vi "AprilTag Target Package Test Code.vi"() -> ()   [LabVIEW 2023]
uses:
  Camera Info.ctl
  State Machine/AprialTag Main Cluster.ctl
  State Machine/AprialTag States.ctl
  <vilib>/vision/Image Controls.llb/IMAQ Image.ctl
  Steam Type.ctl
  Camera Set Up/Event Setup Types.ctl
  <vilib>/Utility/config.llb/Read Key (String).vi
  <vilib>/Utility/config.llb/Write Key (String).vi
  <vilib>/Utility/config.llb/NI_LVConfig.lvlib
panel:
  in  "Main":enum32{"Page 1", "Page 2"}(tab)
  out "Target Pitch":dbl[](array[numeric]) caption="Tag Pitch (deg)" format="%.1f"
  out "Target Roll":dbl[](array[numeric]) caption="Tag Yaw (deg)" format="%.1f"
  out "Tag ID":dbl[](array[numeric]) caption="Tag Number"
  out "Image":T1(plugin-control)
  in  "Camera Name":string="cam0"
  in  "Settings":bool
  in  "Save":bool
  in  "Tools":bool
  out "AprilTag Fps":dbl format="%#.0f"
  out "Distance":dbl[](array[numeric]) caption="Tag Distance (in)" format="%.1f"
  out "Angle":dbl[](array[numeric]) caption="Center Angle (deg)" format="%.1f"
  in  "Home":bool
  in  "FOV":dbl=68.5
  in  "Robot Calibration Cluster":T2={"Camera Height on robot (in)"=9.5, "Camera Angle on the robot (deg)"=2.5, "Camera FOV Top to Bottom View Angle (deg)"=26.5, "Target size (in)"=6.5, "Distance to front of bumper (in)"=9.75} {"Distance to front of bumper (in)" format="%#_13g"; "Target size (in)" format="%#_13g"; "Camera FOV Top to Bottom View Angle (deg)" format="%#_13g"; "Camera Angle on the robot (deg)" format="%#_13g"; "Camera Height on robot (in)" format="%#_13g"}
  # "Edit the camera name to the camera that you are going to use for this target package"
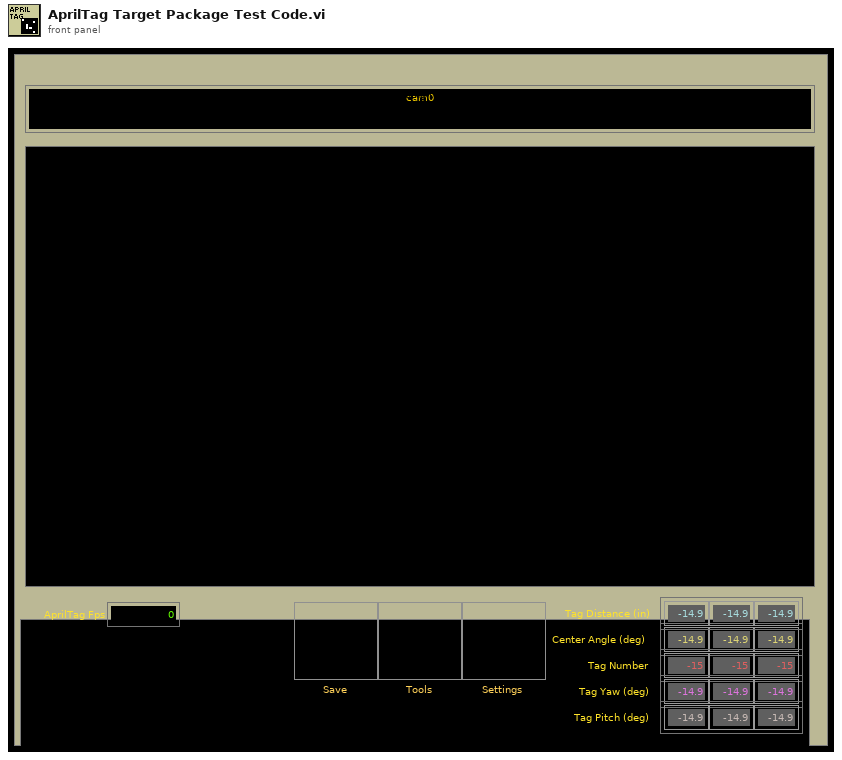
[diagram p1: front panel]
types:
  T1 = typedef "IMAQ Image.ctl" = refnum<image>
  T2 = typedef "Camera Info.ctl" = cluster{"Camera Height on robot (in)":dbl, "Camera Angle on the robot (deg)":dbl, "Camera FOV Top to Bottom View Angle (deg)":dbl, "Target size (in)":dbl, "Distance to front of bumper (in)":dbl}
  T3 = typedef "AprialTag States.ctl" = enum16{"Message Dispatcher", "INI", "Open", "Save", "Exit"}
  T4 = typedef "AprialTag Main Cluster.ctl" = cluster{"AprilTage FIFO":T3[], "Camera Name":string, "AprilTag path":path, "Control Ref's":refnum<vi>[], "Greyscale Mask Image":T1, "Main Image":T1, "Timeout":i32, "EDIT Settings":bool, "Calibration path":path}
  T5 = typedef "Steam Type.ctl" = enum8{"Unknown", "Apriltag", "Algae", "Coral"}
  T6 = typedef "Event Setup Types.ctl" = enum16{"Default", "Camera Loop Started", "Close Settings", "Open Front Panel", "Save Data", "Exit"}
  T7 = typedef "Image Type" = u32
  T8 = cluster{"tag ID":i32, "Center":cluster{"X":dbl, "Y":dbl}, "homography matrix":dbl[], "decision margin":dbl, "Hamming Dist":i32, "corner points":cluster{"X":dbl, "Y":dbl}[], "Tag Family":string}[]
  T9 = typedef "AprilTag Target Fields.ctl" = cluster{"diameter points":cluster{"first point":cluster{"x":dbl, "y":dbl}, "projected point":cluster{"x":dbl, "y":dbl}}, "normalized center":cluster{"x":dbl, "y":dbl}, "Overall Score":dbl, "Distance (ft)":dbl, "Offset Angle":dbl, "Tag corner points":cluster{"X":dbl, "Y":dbl}[], "Tag Center":cluster{"X":dbl, "Y":dbl}, "Tag Yaw":dbl, "Tag Pitch":dbl, "AprilTag Number":i32}
  T10 = typedef "NI_LVConfig.lvlib/Config Data RefNum.ctl" = refnum<k1>
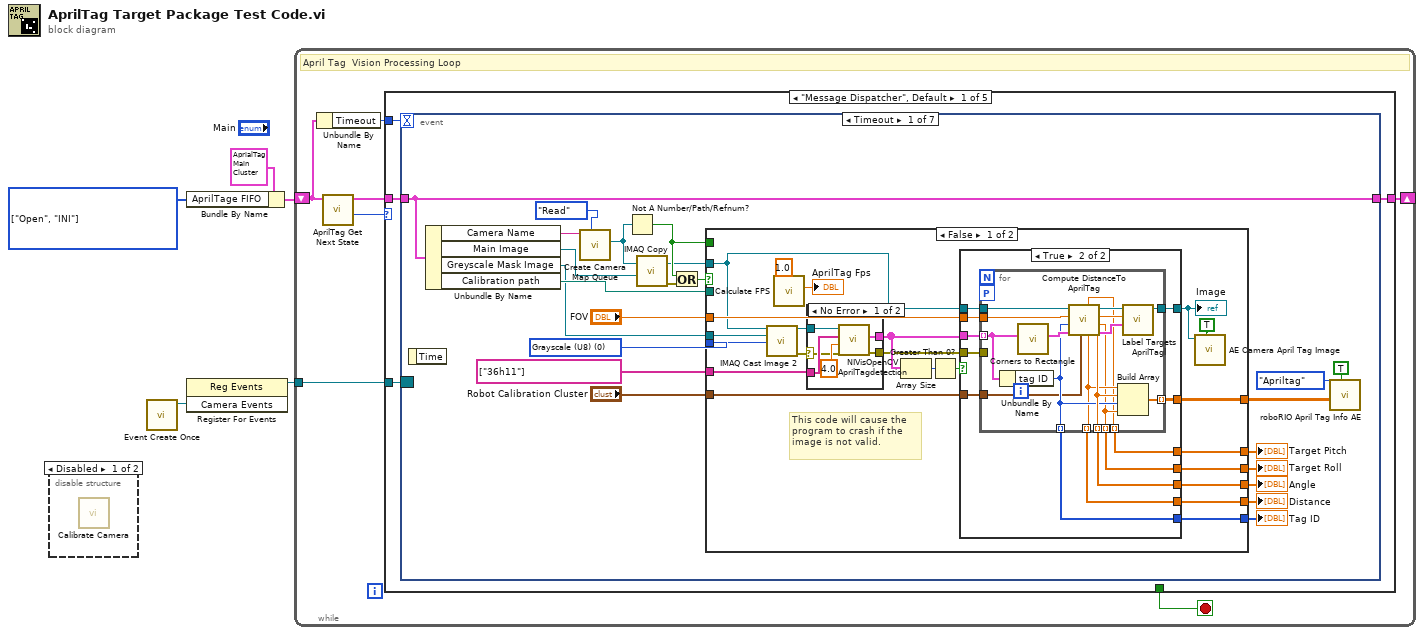
[diagram p0: block diagram]
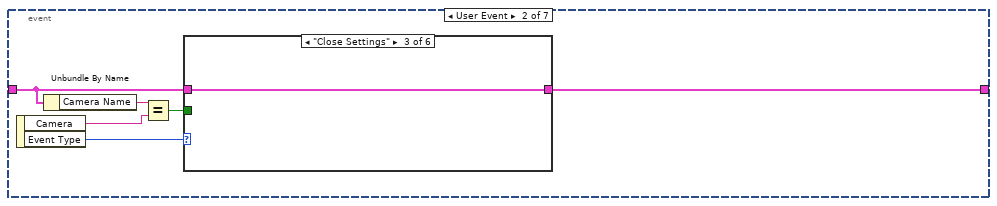
[diagram p6: hidden frame]
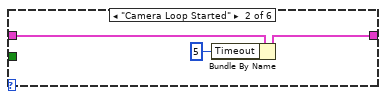
[diagram p8: hidden frame]
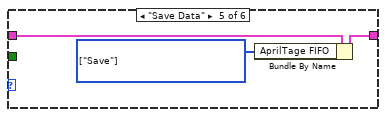
[diagram p10: hidden frame]
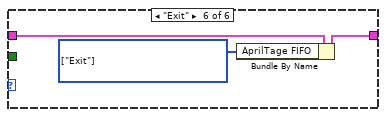
[diagram p11: hidden frame]
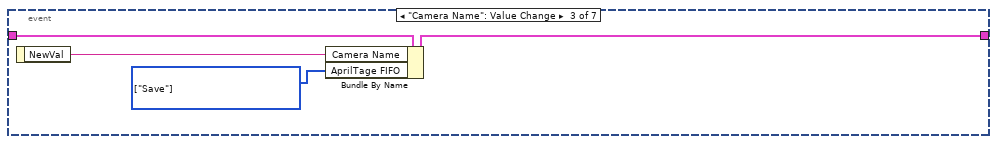
[diagram p12: hidden frame]
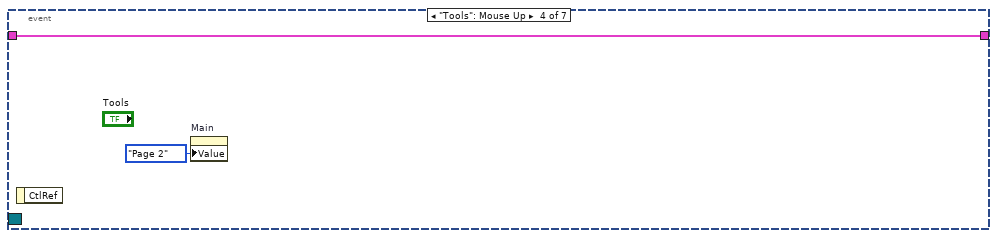
[diagram p13: hidden frame]
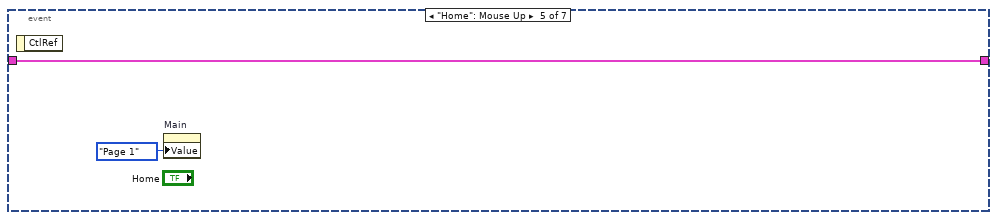
[diagram p14: hidden frame]
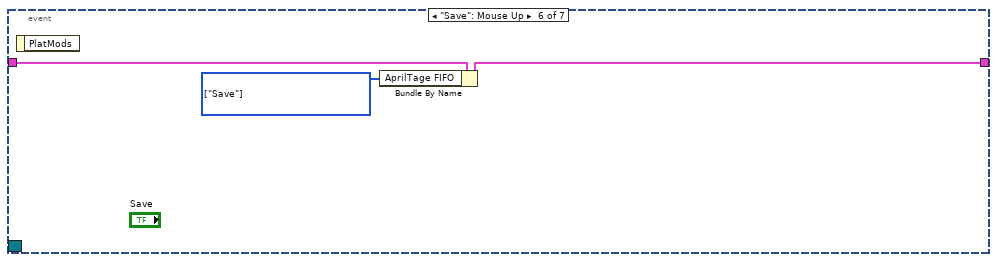
[diagram p15: hidden frame]
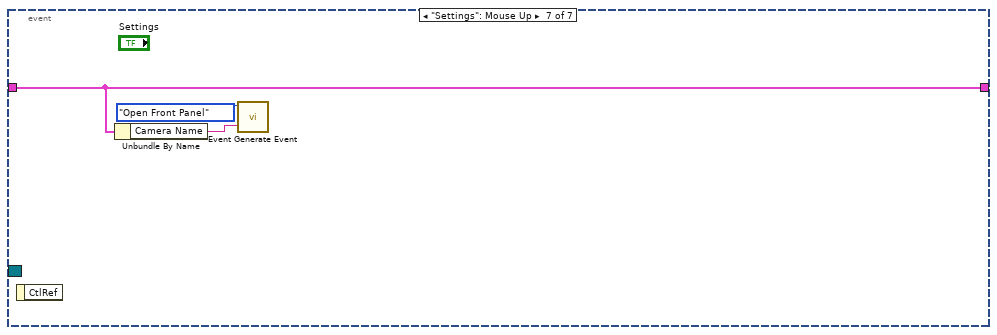
[diagram p16: hidden frame]
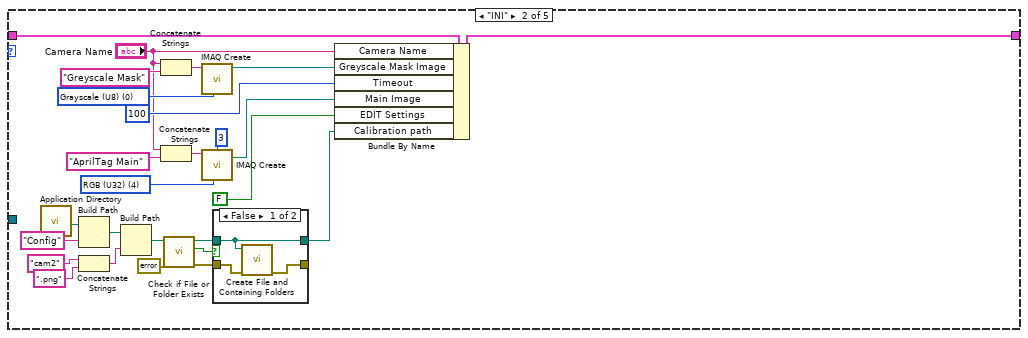
[diagram p17: hidden frame]
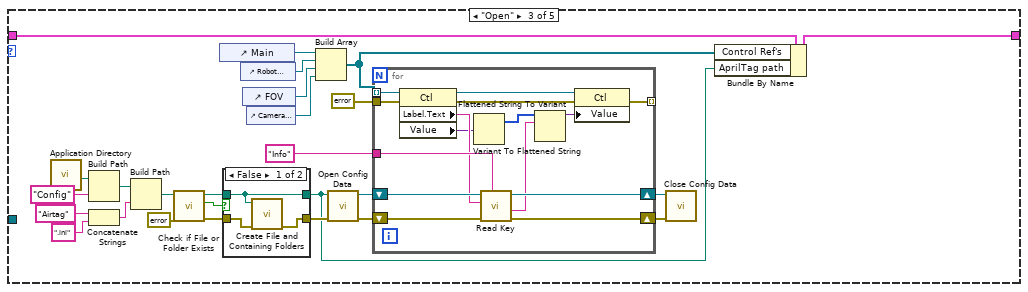
[diagram p19: hidden frame]
diagram:
  w1 = T3[] [enum."Open", enum."INI"] items=["Message Dispatcher", "INI", "Open", "Save", "Exit"] ("AprilTage FIFO")
  n1 = disable-structure shown="Disabled" {
    frame Disabled {
      n2 = call "Calibrate Camera.vi"() -> ()  [unwired: 14 in, 2 out]
    }
    frame Enabled {
    }
  }
  n3 = call "Event Create Once.vi"() -> ("Camera Events"=w5:refnum<user-event>)  [unwired: 10 in, 1 out]
  n4 = Bundle By Name(cluster=T4 {"AprilTage FIFO"=[], "Camera Name"="", "AprilTag path"=path "", "Control Ref's"=[], "Greyscale Mask Image"=refnum, "Main Image"=refnum, "Timeout"=5, "EDIT Settings"=FALSE, "Calibration path"=path ""} ("AprilTag Main Cluster out"), "AprilTage FIFO"=w1) -> (w2:T4)
  n5 = register-events(w5) -> (reference out=w4:refnum<event-registration>)  [unwired: 2 in, 1 out]
  n6 = while {
    tunnel: w4 -> [w12]
    shift-right: [w8] -> _
    shift-left: w2 -> [w6]
    stop <- w11 stop-if-true
    # "April Tag  Vision Processing Loop"
    n7 = Unbundle By Name(w6) -> ("Timeout"=w7:i32)
    n8 = call "AprilTag Get Next State.vi"("AprilTag Main Cluster in"=w6) -> ("Next State"=w9:T3, "AprilTag Main Cluster out"=w10:T4)  [unwired: 9 in]
    n9 = case shown="\"Message Dispatcher\", Default" w9 {
      tunnel: w12 -> [w16 _ _ _ _]
      tunnel: [_ _ _ _ TRUE] -> w11
      tunnel: w10 -> [w14 w153 w170 w208 w225]
      tunnel: [w15 w152 w168 w208 w225] -> w8
      tunnel: w7 -> [w13 _ _ _ _]
      frame "Message Dispatcher", Default {
        n10 = event shown="[0] Timeout" {
          selector: w16 -> [_ _ _ _ _ _ _]
          dyn-events: _ -> [_ _ _ _ _ _ _]
          timeout: w13 -> [_ _ _ _ _ _ _]
          tunnel: w14 -> [w39 w99 w117 w118 w120 w124 w126]
          tunnel: [w39 w101 w116 w118 w120 w123 w126] -> w15
          event Timeout {
            w34 = T7 0 items=["Grayscale (U8)", "Grayscale (I16)", "Grayscale (SGL)", "Complex (CSG)", "RGB (U32)", "HSL (U32)", "RGB (U64)", "Grayscale (U16)"] ("Image Type")
            n11 = event-data() -> ()  [unwired: 1 in, 1 out]
            n12 = Unbundle By Name(w39) -> ("Camera Name"=w23:string, "Main Image"=w17:T1, "Greyscale Mask Image"=w18:T1, "Calibration path"=w35:path)
            n13 = call "Create Camera Map Queue.vi"("Action"=enum16{"Read", "Write"}."Read", "Camera"=w23) -> ("Image out"=w22:T1)  [unwired: 8 in, 1 out]
            n14 = Not A Number/Path/Refnum?(number/path/refnum=w22) -> (NaN/Path/Refnum?=w30:bool)
            n15 = call "IMAQ Copy"("Image Dst"=w17, "Image Src"=w22) -> ("error out"=w20:errorcluster, "Image Dst Out"=w19:T1)  [unwired: 4 in]
            n16 = Or(x=w30, y=w20) -> (x .or. y?=w21:bool)
            n17 = case shown="False" w21 {
              tunnel: w34 -> [w61 _]
              tunnel: string[] ["36h11"] ("Tag Familys") -> [w60 _]
              tunnel: "FOV" -> [w59 _]
              tunnel: "Robot Calibration Cluster" -> [w58 _]
              tunnel: [w48 _] -> w37
              tunnel: w30 -> [_ _]
              tunnel: w35 -> [_ _]
              tunnel: [w46 _] -> w29
              tunnel: [w45 _] -> w28
              tunnel: [w44 _] -> w27
              tunnel: [w43 _] -> w26
              tunnel: [w42 _] -> w25
              tunnel: w19 -> [w41 _]
              tunnel: w18 -> [w40 _]
              frame False {
                # "This code will cause the program to crash if the image is not valid."
                n18 = call "IMAQ Cast Image 2"("Image Src"=w41, "Image Dst"=w40, "Image Type"=w61) -> ("Image Dst Out"=w57:T1, "error out"=w47:errorcluster)  [unwired: 11 in]
                n19 = call "Calculate FPS.vi"("Frames Processed"=1.0) -> ("Fps"=→"AprilTag Fps":dbl)  [unwired: 10 in]
                n20 = case shown="No Error" w47 {
                  selector: w47 -> [w62 w68]
                  tunnel: w60 -> [w67 _]
                  tunnel: w57 -> [w66 _]
                  tunnel: [w65 _] -> w56
                  tunnel: [w64 w68] -> w53
                  frame No Error {
                    n21 = call "NIVisOpenCV AprilTagdetection.vi"("error in (no error)"=w62, "decimate"=4.0, "Tag Familys"=w67, "Image Src"=w66) -> ("error out"=w64:errorcluster, "Detected Tags"=w65:T8)  [unwired: 4 in, 2 out]
                  }
                  frame Error {
                  }
                }
                n22 = Array Size(array=w56) -> (size(s)=w55:i32)
                n23 = Greater Than 0?(x=w55) -> (x > 0?=w54:bool)
                n24 = case shown="True" w54 {
                  tunnel: w41 -> [w69 w81]
                  tunnel: w56 -> [_ w80]
                  tunnel: [w69 w79] -> w52
                  tunnel: w53 -> [_ w78]
                  tunnel: w59 -> [_ w77]
                  tunnel: w58 -> [_ w76]
                  tunnel: [_ w75] -> w48
                  tunnel: [_ w74] -> w46
                  tunnel: [_ w73] -> w45
                  tunnel: [_ w72] -> w44
                  tunnel: [_ w71] -> w43
                  tunnel: [_ w70] -> w42
                  frame False {
                  }
                  frame True {
                    n25 = for {
                      tunnel: w80 -> [w93] mode=indexing
                      tunnel: w81 -> [w94]
                      tunnel: [w95] -> w79
                      tunnel: w78 -> [_]
                      tunnel: [w87] -> w72 mode=indexing
                      tunnel: [w85] -> w70 mode=indexing
                      tunnel: [w89] -> w71 mode=indexing
                      tunnel: w77 -> [w88]
                      tunnel: w76 -> [w86]
                      tunnel: [w84] -> w73 mode=indexing
                      tunnel: [w83] -> w75 mode=indexing
                      tunnel: [w82] -> w74 mode=indexing
                      workers-P: _ -> [_]
                      n26 = Unbundle By Name(w93) -> ("tag ID"=w87:i32)
                      n27 = call "Corners to Rectangle.vi"("tag info"=w93) -> ("output cluster"=w92:T9)  [unwired: 10 in]
                      n28 = call "Compute DistanceTo AprilTag.vi"("Robot Calibration Cluster"=w86, "results"=w92, "AprilTag Number"=w87, "FOV Left to Right (deg)"=w88, "Image Src"=w94) -> ("results out"=w91:T9, "Target Yaw (deg)"=w84:dbl, "Offset Angle"=w89:dbl, "Image Dst Out"=w90:T1, "Distance from target (in)"=w85:dbl, "Target Pitch (deg)"=w82:dbl)  [unwired: 1 in]
                      n29 = Build Array(w85, w89, w87, w84) -> (w83:dbl[])
                      n30 = call "Label Targets AprilTagl.vi"("results"=w91, "Angle"=w89, "Image in"=w90) -> ("Image out"=w95:T1)  [unwired: 8 in]
                    }
                  }
                }
                "Image" <- w52
                n31 = call "AE Camera April Tag Image.vi"("Update"=TRUE, "Ball Image in"=w52) -> ()  [unwired: 9 in, 1 out]
              }
              frame True {
              }
            }
            "Distance" <- w25
            "Angle" <- w26
            "Tag ID" <- w27
            "Target Roll" <- w28
            "Target Pitch" <- w29
            n32 = call "roboRIO April Tag Info AE.vi"("Update"=TRUE, "Info in"=w37, "Stream Type"=Steam_Type."Apriltag") -> ()  [unwired: 8 in, 1 out]
          }
          event User Event {
            n33 = event-data() -> ("Camera"=w97:string, "Event Type"=w100:T6)  [unwired: 1 in]
            n34 = Unbundle By Name(w99) -> ("Camera Name"=w98:string)
            n35 = Equal?(x=w98, y=w97) -> (x = y?=w96:bool)
            n36 = case shown="\"Close Settings\"" w100 {
              tunnel: w99 -> [w102 w105 w106 w107 w110 w113]
              tunnel: [w102 w104 w106 w107 w109 w112] -> w101
              tunnel: w96 -> [_ _ _ _ _ _]
              frame "Default" {
              }
              frame "Camera Loop Started" {
                n37 = Bundle By Name(cluster=w105, "Timeout"=5) -> (w104:T4)
              }
              frame "Close Settings" {
              }
              frame "Open Front Panel" {
              }
              frame "Save Data" {
                w108 = T3[] [enum."Save"] items=["Message Dispatcher", "INI", "Open", "Save", "Exit"] ("AprilTage FIFO")
                n38 = Bundle By Name(cluster=w110, "AprilTage FIFO"=w108) -> (w109:T4)
              }
              frame "Exit" {
                w111 = T3[] [enum."Exit"] items=["Message Dispatcher", "INI", "Open", "Save", "Exit"] ("AprilTage FIFO")
                n39 = Bundle By Name(cluster=w113, "AprilTage FIFO"=w111) -> (w112:T4)
              }
            }
          }
          event "Camera Name": Value Change {
            w115 = T3[] [enum."Save"] items=["Message Dispatcher", "INI", "Open", "Save", "Exit"] ("AprilTage FIFO")
            n40 = event-data() -> ("NewVal"=w114:string)  [unwired: 1 in]
            n41 = Bundle By Name(cluster=w117, "Camera Name"=w114, "AprilTage FIFO"=w115) -> (w116:T4)
          }
          event "Tools": Mouse Up {
            n42 = event-data() -> ()  [unwired: 1 in, 1 out]
            n43 = property on="Main" class="TabCtl (strict)"("Value"=enum32{"Page 1", "Page 2"}."Page 2" ("Main")) -> ()  [unwired: 2 in, 2 out]
          }
          event "Home": Mouse Up {
            n44 = event-data() -> ()  [unwired: 1 in, 1 out]
            n45 = property on="Main" class="TabCtl (strict)"("Value"=enum32{"Page 1", "Page 2"}."Page 1" ("Main")) -> ()  [unwired: 2 in, 2 out]
          }
          event "Save": Mouse Up {
            w122 = T3[] [enum."Save"] items=["Message Dispatcher", "INI", "Open", "Save", "Exit"] ("AprilTage FIFO")
            n46 = event-data() -> ()  [unwired: 1 in, 1 out]
            n47 = Bundle By Name(cluster=w124, "AprilTage FIFO"=w122) -> (w123:T4)
          }
          event "Settings": Mouse Up {
            n48 = event-data() -> ()  [unwired: 1 in, 1 out]
            n49 = Unbundle By Name(w126) -> ("Camera Name"=w125:string)
            n50 = call "Event Generate Event.vi"("Camera Name"=w125, "Event Type"=Event_Setup_Types."Open Front Panel") -> ()  [unwired: 10 in]
          }
        }
      }
      frame "INI" {
        w146 = T7 4 items=["Grayscale (U8)", "Grayscale (I16)", "Grayscale (SGL)", "Complex (CSG)", "RGB (U32)", "HSL (U32)", "RGB (U64)", "Grayscale (U16)"] ("Image Type")
        w149 = T7 0 items=["Grayscale (U8)", "Grayscale (I16)", "Grayscale (SGL)", "Complex (CSG)", "RGB (U32)", "HSL (U32)", "RGB (U64)", "Grayscale (U16)"] ("Image Type")
        n51 = call <vilib>:"Application Directory.vi"() -> ("Application Directory"=w137:path)
        n52 = Build Path(base path=w137, name or relative path="Config") -> (appended path=w135:path)
        n53 = Concatenate Strings("cam2" ("string"), ".png" ("name or relative path")) -> (w139:string)
        n54 = Build Path(base path=w135, name or relative path=w139) -> (appended path=w134:path)
        n55 = Concatenate Strings("Camera Name", "Greyscale Mask" ("string")) -> (w150:string)
        n56 = Concatenate Strings("Camera Name", "AprilTag Main" ("string")) -> (w145:string)
        n57 = call <vilib>:"Check if File or Folder Exists.vi"("error in (no error)"=errorcluster {"status"=FALSE, "code"=0, "source"=""}, "path"=w134) -> ("error out"=w131:errorcluster, "file or folder exists?"=w132:bool, "dup path"=w133:path)  [unwired: 7 in]
        n58 = call "IMAQ Create"("Image Name"=w150, "Image Type"=w149) -> ("New Image"=w148:T1)  [unwired: 2 in, 2 out]
        n59 = call "IMAQ Create"("Border Size"=3, "Image Name"=w145, "Image Type"=w146) -> ("New Image"=w143:T1)  [unwired: 1 in, 2 out]
        n60 = case shown="False" w132 {
          tunnel: [w156 w157] -> _
          tunnel: w133 -> [w155 w158]
          tunnel: [w155 w158] -> w128
          tunnel: w131 -> [w154 w157]
          frame False {
            n61 = call <vilib>:"Create File and Containing Folders.vi"("error in (no error)"=w154, "file path"=w155) -> ("error out"=w156:errorcluster)  [unwired: 8 in, 1 out]
          }
          frame True {
          }
        }
        n62 = Bundle By Name(cluster=w153, "Camera Name"="Camera Name", "Greyscale Mask Image"=w148, "Timeout"=100, "Main Image"=w143, "EDIT Settings"=FALSE, "Calibration path"=w128) -> (w152:T4)
      }
      frame "Open" {
        n63 = call <vilib>:"Application Directory.vi"() -> ("Application Directory"=w173:path)
        n64 = Build Path(base path=w173, name or relative path="Config") -> (appended path=w171:path)
        n65 = Concatenate Strings("Airtag" ("string"), ".ini" ("name or relative path")) -> (w184:string)
        n66 = Build Path(base path=w171, name or relative path=w184) -> (appended path=w164:path)
        n67 = call <vilib>:"Check if File or Folder Exists.vi"("error in (no error)"=errorcluster {"status"=FALSE, "code"=0, "source"=""}, "path"=w164) -> ("error out"=w160:errorcluster, "file or folder exists?"=w162:bool, "dup path"=w163:path)  [unwired: 7 in]
        n68 = control-ref of="Main"() -> (w179:refnum<vi>)
        n69 = case shown="False" w162 {
          tunnel: [w187 w188] -> w174
          tunnel: w163 -> [w186 w189]
          tunnel: [w186 w189] -> w161
          tunnel: w160 -> [w185 w188]
          frame False {
            n70 = call <vilib>:"Create File and Containing Folders.vi"("error in (no error)"=w185, "file path"=w186) -> ("error out"=w187:errorcluster)  [unwired: 8 in, 1 out]
          }
          frame True {
          }
        }
        n71 = control-ref of="Robot Calibration Cluster"() -> (w178:refnum<vi>)
        n72 = control-ref of="FOV"() -> (w177:refnum<vi>)
        n73 = control-ref of="Camera Name"() -> (w169:refnum<vi>)
        n74 = Build Array(w179, w178, w177, w169) -> (w167:refnum<vi>[])
        n75 = call <vilib>:"Open Config Data.vi"("error in (no error)"=w174, "configuration file path"=w161) -> ("error out"=w180:errorcluster, "refnum"=w183:T10)  [unwired: 7 in, 1 out]
        n76 = for {
          tunnel: "Info" ("Camera Name") -> [w201]
          tunnel: w167 -> [w199] mode=indexing
          shift-right: [w203] -> w182
          shift-left: w183 -> [w204]
          shift-right: [w202] -> w181
          shift-left: w180 -> [w200]
          tunnel: [w194] -> _ mode=indexing
          tunnel: errorcluster {"status"=FALSE, "code"=0, "source"=""} ("error out") -> [w193]
          n77 = property class="Ctl"(reference=w199, error in=w193) -> (reference out=w197:refnum<vi>, error out=w195:errorcluster, "Label.Text"=w198:string, "Value"=w191:variant)
          n78 = Variant To Flattened String(Variant=w191) -> (1:w190:i16[])  [unwired: 1 out]
          n79 = call-poly <vilib>:"Read Key.vi"("section"=w201, "error in (no error)"=w200, "key"=w198, "refnum"=w204) -> ("error out"=w202:errorcluster, "value"=w196:string, "refnum out"=w203:T10)  [unwired: 4 in, 1 out]
          n80 = Flattened String To Variant(6:w196, 7:w190) -> (3:w192:variant)  [unwired: 1 in, 1 out]
          n81 = property class="Ctl"(reference=w197, error in=w195, "Value"=w192) -> (error out=w194:errorcluster)  [unwired: 1 out]
        }
        n82 = call <vilib>:"Close Config Data.vi"("error in (no error)"=w181, "refnum"=w182) -> ()  [unwired: 8 in, 2 out]
        n83 = Bundle By Name(cluster=w170, "Control Ref's"=w167, "AprilTag path"=w161) -> (w168:T4)
      }
      frame "Save" {
        n84 = Unbundle By Name(w208) -> ("Control Ref's"=w206:refnum<vi>[], "AprilTag path"=w207:path)
        n85 = call <vilib>:"Open Config Data.vi"("configuration file path"=w207) -> ("error out"=w209:errorcluster, "refnum"=w212:T10)  [unwired: 8 in, 1 out]
        n86 = for {
          tunnel: "Info" ("Camera Name") -> [w218]
          shift-right: [w221] -> w211
          shift-left: w212 -> [w222]
          shift-right: [w220] -> w210
          shift-left: w209 -> [w219]
          tunnel: w206 -> [w213] mode=indexing
          n87 = property class="Ctl"(reference=w213, error in=w219) -> (error out=w215:errorcluster, "Label.Text"=w217:string, "Value"=w216:variant)  [unwired: 1 out]
          n88 = Variant To Flattened String(Variant=w216) -> (data string=w214:string)  [unwired: 1 out]
          n89 = call-poly <vilib>:"Write Key.vi"("section"=w218, "error in (no error)"=w215, "value"=w214, "key"=w217, "refnum"=w222) -> ("error out"=w220:errorcluster, "refnum out"=w221:T10)  [unwired: 4 in, 1 out]
        }
        n90 = call <vilib>:"Close Config Data.vi"("error in (no error)"=w210, "refnum"=w211) -> ()  [unwired: 8 in, 2 out]
      }
      frame "Exit" {
        n91 = Unbundle By Name(w225) -> ("Greyscale Mask Image"=w224:T1, "Main Image"=w223:T1)
        n92 = call "IMAQ Dispose"("Image"=w224) -> ()  [unwired: 5 in, 1 out]
        n93 = call "IMAQ Dispose"("Image"=w223) -> ()  [unwired: 5 in, 1 out]
      }
    }
  }
